vi "Move Splitter.vi"(6 "Loop Number (16)":i32=16, 8 "error in (no error)":errorcluster, 9 "Splitter Position":i32, 10 "Splitter Name":string, 11 "IViewManager in":refnum<class "IViewManager.lvclass">) -> (0 "error out":errorcluster, 3 "IViewManager out":refnum<class "IViewManager.lvclass">)   [LabVIEW 2020, in "IViewManager.lvlib" / "IViewManager.lvclass"]
uses:
  <vilib>/gpm_packages/@cs/mva-viewable/Source/IViewManager/IViewManager/IViewManager.lvclass
  <vilib>/gpm_packages/@cs/mva-viewable/Source/IViewManager/IViewManager/IViewManager.lvclass/IViewManager.ctl
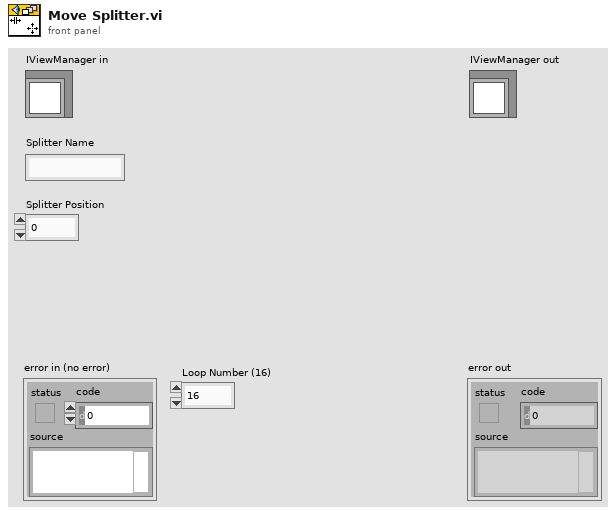
[diagram p1: front panel]
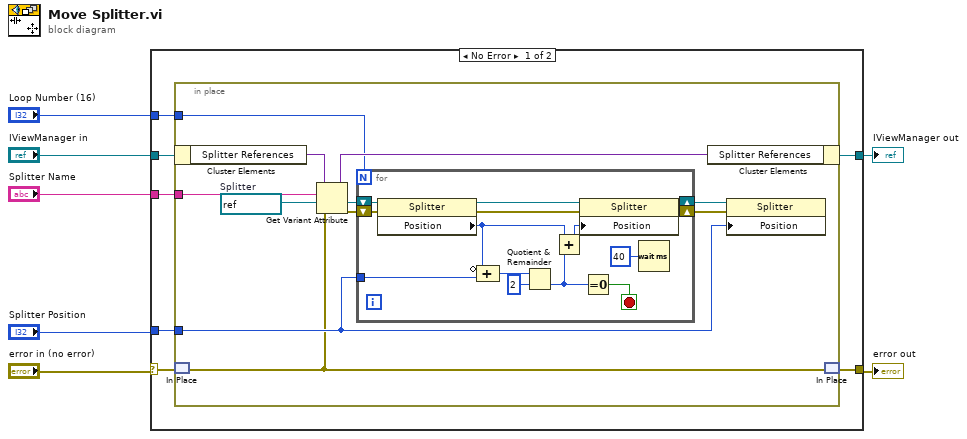
[diagram p0: block diagram]
diagram:
  n1 = case shown="No Error" "error in (no error)" {
    selector: "error in (no error)" -> [w10 w41]
    tunnel: "IViewManager in" -> [w14 w40]
    tunnel: "Splitter Name" -> [w13 _]
    tunnel: "Splitter Position" -> [w12 _]
    tunnel: "Loop Number (16)" -> [w11 _]
    tunnel: [w9 w41] -> w1
    tunnel: [w8 w40] -> w2
    frame No Error {
      n2 = in-place {
        in-place-border: w13 -> [w24]
        in-place-border: w12 -> [w17]
        in-place-border: w11 -> [w16]
        w23 = refnum<vi> refnum  # Splitter
        n3 = in-place-cluster #1(w14) -> ("Splitter References"=w25:variant)
        n4 = in-place-match #2(w10) -> (w15:errorcluster)
        n5 = Get Variant Attribute(Variant=w25, name=w24, default value (empty Variant)=w23, error in=w15) -> (duplicate Variant=w22:variant, value=w19:refnum<vi>, error out=w18:errorcluster)  [unwired: 1 out]
        n6 = for {
          N: w16 -> [_]
          shift-right: [w37] -> w20
          shift-left: w19 -> [w39]
          shift-right: [w30] -> w21
          shift-left: w18 -> [w38]
          tunnel: w17 -> [w26]
          stop <- w29 stop-if-true
          n7 = property class="Splitter"(reference=w39, error in=w38) -> (reference out=w35:refnum<vi>, error out=w36:errorcluster, "Position"=w27:i32)
          n8 = Compound Arithmetic op=ADD(invert w27, w26) -> (w33:i32)
          n9 = Quotient & Remainder(x=w33, y=2) -> (floor(x/y)=w31:i32)  [unwired: 1 out]
          n10 = Add(x=w27, y=w31) -> (x+y=w34:i32)
          n11 = property class="Splitter"(reference=w35, error in=w36, "Position"=w34) -> (reference out=w37:refnum<vi>, error out=w30:errorcluster)
          n12 = Equal To 0?(x=w31) -> (x = 0?=w29:bool)
          n13 = Wait (ms)(milliseconds to wait=u32 40) -> ()  [unwired: 1 out]
        }
        n14 = in-place-cluster #1("Splitter References"=w22) -> (w8:refnum<class "IViewManager.lvclass">)
        n15 = property class="Splitter"(reference=w20, error in=w21, "Position"=w17) -> ()  [unwired: 2 out]
        n16 = in-place-match #2(w15) -> (w9:errorcluster)
      }
    }
    frame Error {
    }
  }
  "error out" <- w1
  "IViewManager out" <- w2
